vi "Main.vi"(10 "COM port name":refnum<visa-resource-name>, 11 "Module Admin":refnum<class "Delacor_lib_QMH_Cloneable Module Admin.lvclass">) -> ()   [LabVIEW 2018, in "CE14_v2.lvlib"]
doc: "This template is based off of the Queued Message Handler design pattern and the Queued Message Handler project template that ships with LabVIEW.\n\nThe main difference is that the queue is private to this module and communication between modules is performed via Broadcast and Request events.\n\nRequest events are wrapped in public API methods and are handled in the Event Handling Loop (EHL) of this VI. Any module can register for Broadcast events sent by this module. The EHL generates messages based on user interface actions.\n\nThe Message Handling Loop (MHL) processes messages generated by the EHL, or by other messages. The messages are string values, so new messages can be added easily to the Message Cases case structure in the MHL. Each message cluster can also provide an optional value for Message Data, which is a variant that can be converted to whatever message-specific data is required.\n_____\nBased on DQMH Project Template 6.0.0.91."
uses:
  CE14_v2.lvlib
  <vilib>/Delacor/Delacor QMH/Libraries/Cloneable Module Admin_class/Delacor_lib_QMH_Cloneable Module Admin.lvclass
  C:/Program Files (x86)/National Instruments/LabVIEW 2018/vi.lib/Delacor/Delacor QMH/Libraries/Module Admin_class/Delacor_lib_QMH_Module Admin.lvclass
  <vilib>/Delacor/Delacor QMH/Libraries/Message Queue_class/Delacor_lib_QMH_Message Queue.lvclass/Delacor_lib_QMH_Message Queue.ctl
  Module Data--cluster.ctl
  <vilib>/Delacor/Delacor QMH/Libraries/Cloneable Module Admin_class/Delacor_lib_QMH_Cloneable Module Admin.lvclass/Delacor_lib_QMH_Cloneable Module Admin.ctl
  Stop Argument--cluster.ctl
  <vilib>/Delacor/Delacor QMH/Libraries/Module Admin_class/Delacor_lib_QMH_Module Admin.lvclass/Delacor_lib_QMH_Module Admin.ctl
  CE14.CheckConnected Argument--cluster.ctl
  CE14.CheckConnected (Reply Payload)--cluster.ctl
  Read AC parameters Argument--cluster.ctl
  Connect to CE14 Argument--cluster.ctl
  <vilib>/Utility/miscctls.llb/LVPointTypeDef.ctl
  Instrument Drivers/LVdriver_CE14(eMIC)/type defs/CE14.data.ctl
  <vilib>/Delacor/Delacor QMH/Libraries/Message Queue_class/Delacor_lib_QMH_Enqueue Message (Single).vi
  <vilib>/Delacor/Delacor QMH/Libraries/Cloneable Module Admin_class/Delacor_lib_QMH_Get Module ID.vi
  <vilib>/Delacor/Delacor QMH/Libraries/Module Admin_class/Delacor_lib_QMH_Get External Launch.vi
  <vilib>/Utility/error.llb/Error Cluster From Error Code.vi
  <vilib>/ErrorRing/Error Ring.xnode
  <vilib>/Delacor/Delacor QMH/Libraries/Message Queue_class/Delacor_lib_QMH_Message Queue.lvclass
  Instrument Drivers/LVdriver_CE14(eMIC)/CE14_eMIC.lvlib
panel:
  out "Frequency":dbl
  out "connected":bool
  out "error out":errorcluster
  out "Status":string
  in  "Simulate EHL Error":bool
  in  "Simulate MHL Error":bool
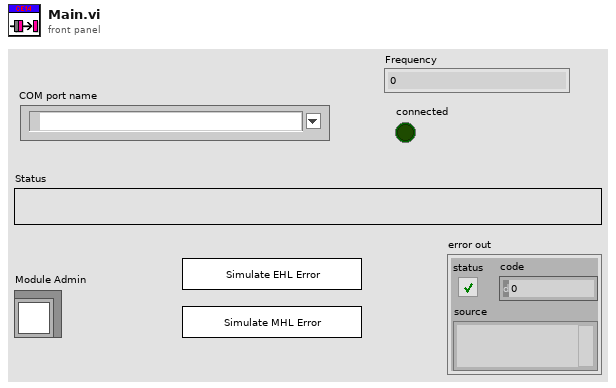
[diagram p1: front panel]
types:
  T1 = typedef "CE14_v2.lvlib/Request Events--cluster.ctl" = cluster{"Stop Module":refnum<user-event>, "Show Panel":refnum<user-event>, "Hide Panel":refnum<user-event>, "Show Diagram":refnum<user-event>, "Get Module Execution Status":refnum<user-event>, "CE14.CheckConnected":refnum<user-event>, "Read AC parameters":refnum<user-event>, "Connect to CE14":refnum<user-event>, "Stop helper loop":refnum<user-event>, "Start Helper Loop":refnum<user-event>}
  T2 = typedef "CE14_v2.lvlib/Module Data--cluster.ctl" = cluster{"Status":string, "VISA resource name":refnum<visa-resource-name>, "connected":bool}
  T3 = enum32{"invalid lock state", "Not Locked", "Locked (No Password)", "Password-protected"}
  T4 = typedef "CE14_v2.lvlib/Stop Argument--cluster.ctl" = cluster{"Module ID":i32, "Origin":string, "Exit via Stop Module Req?":bool, "Wait for Module to stop?":bool}
  T5 = typedef "CE14_v2.lvlib/CE14.CheckConnected Argument--cluster.ctl" = cluster{"Module ID":i32, "Wait Notifier":refnum<notifier>, "wait for reply":bool}
  T6 = typedef "CE14_v2.lvlib/Read AC parameters Argument--cluster.ctl" = cluster{"Module ID":i32, "Boolean":bool}
  T7 = typedef "CE14_v2.lvlib/Connect to CE14 Argument--cluster.ctl" = cluster{"Module ID":i32, "Boolean":bool}
  T8 = typedef "LVPointTypeDef.ctl" = cluster{"Horizontal":i16, "Vertical":i16}
  T9 = enum32{"Invalid", "Standard", "Closed", "Hidden", "Minimized", "Maximized"}
  T10 = typedef "CE14_v2.lvlib/CE14.CheckConnected (Reply Payload)--cluster.ctl" = cluster{"Success":bool, "CE14.CheckConnected_error":errorcluster}
  T11 = typedef "CE14_eMIC.lvlib/CE14.data.ctl" = cluster{"string":string, "float":dbl, "Name":string}
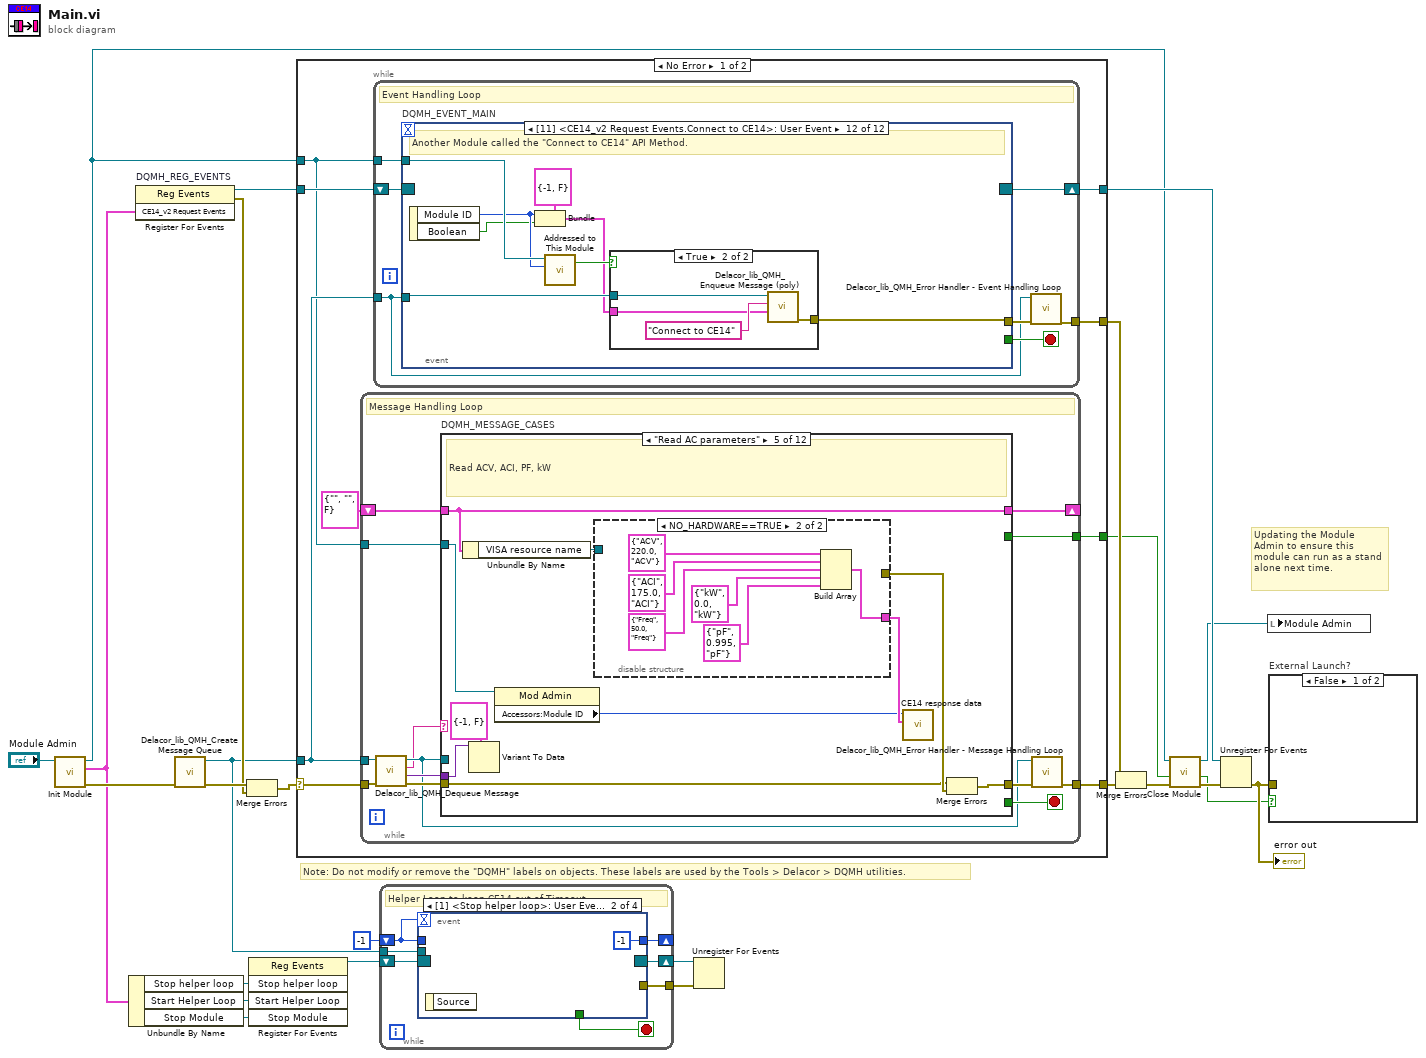
[diagram p0: block diagram]
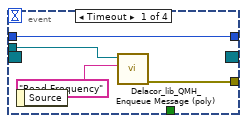
[diagram p2: hidden frame]
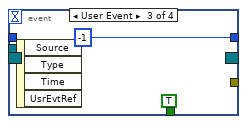
[diagram p3: hidden frame]
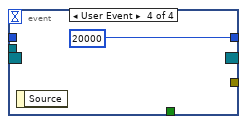
[diagram p4: hidden frame]
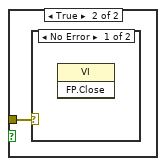
[diagram p5: hidden frame]
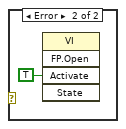
[diagram p6: hidden frame]
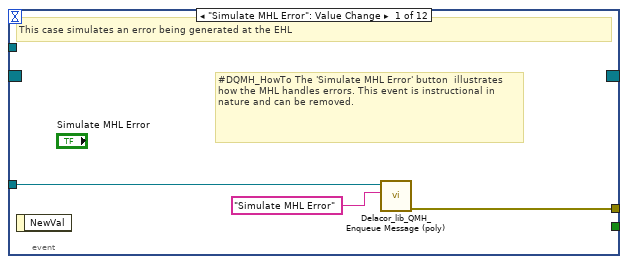
[diagram p7: hidden frame]
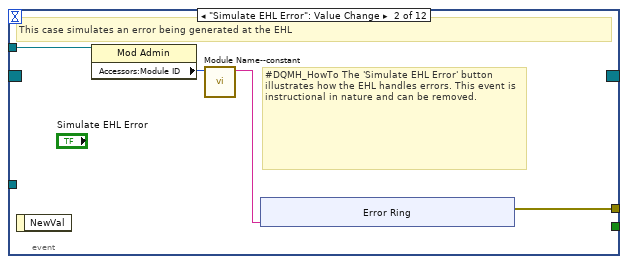
[diagram p8: hidden frame]
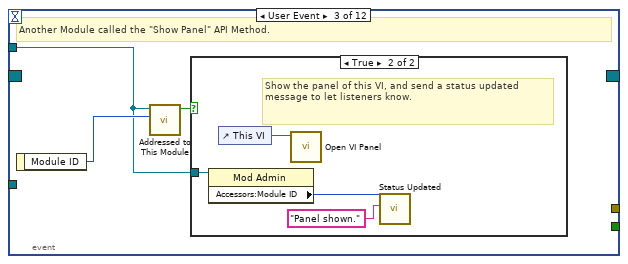
[diagram p9: hidden frame]
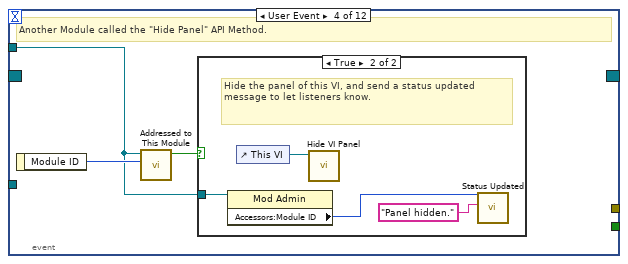
[diagram p11: hidden frame]
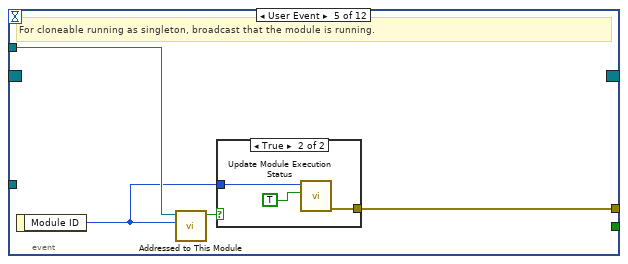
[diagram p13: hidden frame]
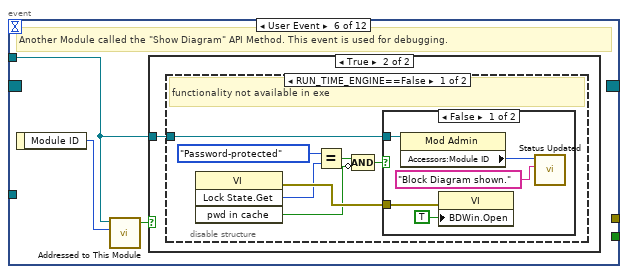
[diagram p15: hidden frame]
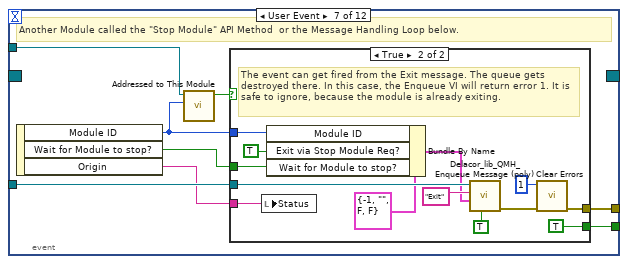
[diagram p19: hidden frame]
diagram:
  # "Note: Do not modify or remove the \"DQMH\" labels on objects. These labels are used by the Tools > Delacor > DQMH utilities."
  # "Updating the Module Admin to ensure this module can run as a stand alone next time."
  n1 = call "Init Module.vi"("Cloneable Module Admin in"="Module Admin") -> ("error out"=w22:errorcluster, "CE14_v2 Request Events"=w8:T1, "Cloneable Module Admin out"=w14:refnum<class "Delacor_lib_QMH_Cloneable Module Admin.lvclass">)  [unwired: 8 in]
  n2 = Unbundle By Name(w8) -> ("Stop helper loop"=w5:refnum<user-event>, "Start Helper Loop"=w4:refnum<user-event>, "Stop Module"=w3:refnum<user-event>)
  n3 = register-events "DQMH_REG_EVENTS"(w8) -> (reference out=w10:refnum<event-registration>, error out=w17:errorcluster)  [unwired: 2 in]
  n4 = call <vilib>:"Delacor_lib_QMH_Create Message Queue.vi"("error in"=w22) -> ("error out"=w19:errorcluster, "Message Queue"=w9:refnum<class "Delacor_lib_QMH_Message Queue.lvclass">)  [unwired: 9 in]
  n5 = Merge Errors(w19, w17) -> (w18:errorcluster)
  n6 = register-events(w5, w4, w3) -> (reference out=w7:refnum<event-registration>)  [unwired: 2 in, 1 out]
  n7 = case shown="No Error" w18 {
    selector: w18 -> [w32 w345]
    tunnel: [w34 w344] -> w23
    tunnel: [w31 w352] -> w16
    tunnel: w10 -> [w29 w352]
    tunnel: w9 -> [w28 w343]
    tunnel: [w33 _] -> w24
    tunnel: w14 -> [w27 w348]
    tunnel: [w26 _] -> w12
    frame No Error {
      n8 = while {
        tunnel: w28 -> [w168]
        shift-right: [w173] -> _
        shift-left: T2 {"Status"="", "VISA resource name"="", "connected"=FALSE} ("Data Cluster") -> [w174]
        tunnel: w32 -> [w169]
        tunnel: [w175] -> w34
        tunnel: w27 -> [w171]
        tunnel: [w170] -> w26
        stop <- w172 stop-if-true
        # "Message Handling Loop"
        n9 = call-dynamic "Delacor_lib_QMH_Dequeue Message.vi"("error in"=w169, "Message Queue in"=w168) -> ("error out"=w166:errorcluster, "Message Data"=w167:variant, "Message"=w164:string, "Message Queue out"=w165:refnum<class "Delacor_lib_QMH_Message Queue.lvclass">)  [unwired: 6 in]
        n10 = case "DQMH_MESSAGE_CASES" shown="\"Read AC parameters\"" w164 {
          selector: w164 -> [_ _ _ _ _ _ _ _ _ _ _ w331]
          tunnel: [w195 w199 w205 w217 w231 w266 w274 w276 w284 w299 w322 w333] -> w176
          tunnel: w174 -> [w179 w200 w203 w220 w237 w268 w275 w277 w283 w297 w313 w332]
          tunnel: [w188 w200 w204 w220 w237 w268 w275 w277 w283 w297 w313 w332] -> w173
          tunnel: [_ _ _ _ _ _ _ _ _ _ w320 _] -> w172
          tunnel: w167 -> [_ _ w209 w227 w239 _ _ _ w282 _ w318 _]
          tunnel: w171 -> [w184 _ _ w216 w233 _ _ _ w281 w295 w308 w329]
          tunnel: [_ _ _ _ _ _ _ _ _ _ w316 _] -> w170
          tunnel: w166 -> [_ w199 w201 w218 w230 w265 w274 w276 _ _ _ _]
          tunnel: w165 -> [_ _ _ _ _ _ _ _ w278 _ w311 _]
          frame "Initialize" {
            w181 = "Initial Message" ("Initial Message")
            # "Initialize - Any operation that needs to be done before the module can receive messages. Synchronize Caller Events.vi will inform Start Module.vi that the module has launched and is ready to receive messages. Module Did Init.vi will broadcast that the module initialized."
            n11 = call "Synchronize Caller Events.vi"("Module Admin"=w184) -> ("error out"=w196:errorcluster, "Module Admin out"=w183:refnum<class "Delacor_lib_QMH_Cloneable Module Admin.lvclass">)  [unwired: 9 in]
            n12 = property class="Mod Admin"(reference=w183) -> ("Accessors:Module ID"=w186:i32, "Accessors:External Launch"=w185:bool)  [unwired: 1 in, 2 out]
            n13 = property on="Pane" class="Pane"("Origin"=T8 {"Horizontal"=0, "Vertical"=0}) -> ()  [unwired: 2 in, 2 out]
            n14 = Bundle By Name(cluster=w179, "VISA resource name"="COM port name") -> (w180:T2)
            n15 = call "Module Name--constant.vi"("Module ID"=w186) -> ("Module Name"=w192:string)  [unwired: 10 in]
            n16 = property class="VI"("Front Panel.Title"=w192) -> (reference out=w194:refnum<vi>, error out=w198:errorcluster)  [unwired: 2 in]
            n17 = Select(t=T9."Hidden" ("State"), s=w185, f=T9."Standard" ("State")) -> (s? t:f=w189:T9)
            n18 = invoke class="VI" method="FP.Open"(reference=w194, error in=w198, "State"=w189) -> (reference out=w193:refnum<vi>, error out=w197:errorcluster)  [unwired: 2 in, 3 out]
            n19 = call "Module Name--constant.vi"("Module ID"=w186) -> ("Module Name"=w187:string)  [unwired: 10 in]
            n20 = Bundle By Name(cluster=w180, "Status"=w181) -> (w188:T2)
            n21 = invoke class="VI" method="FP.Center"(reference=w193, error in=w197) -> ()  [unwired: 1 in, 3 out]
            n22 = call "Module Did Init.vi"("error in (no error)"=w196, "Initialized?"=TRUE, "Origin"=w187, "Module ID"=w186) -> ("error out"=w195:errorcluster)  [unwired: 7 in]
            "Status" <- w181
          }
          frame "---Module Specific---", Default {
            # "Separator -- The following cases handle messages specific to this Module."
          }
          frame "Connect to CE14" {
            # "Open COM and ShakeHand"
            n23 = Unbundle By Name(w203) -> ("VISA resource name"=w207:refnum<visa-resource-name>)
            n24 = Variant To Data(type=T7 {"Module ID"=-1, "Boolean"=FALSE} ("Connect to CE14 Argument"), Variant=w209) -> ()  [unwired: 1 in, 2 out]
            n25 = disable-structure shown="NO_HARDWARE==TRUE" {
              disable-tunnel: w207 -> [w212 _]
              disable-tunnel: [w211 _] -> w206
              disable-tunnel: [w210 TRUE] -> w202
              frame condition #0 {
                n26 = call "CE14.open handshake(subVI).vi"("VISA resource name"=w212) -> ("error out"=w211:errorcluster, "success"=w210:bool)  [unwired: 7 in, 2 out]
              }
              frame condition #1 (active) {
              }
            }
            "connected" <- w202
            n27 = Bundle By Name(cluster=w203, "connected"=w202) -> (w204:T2)
            n28 = Merge Errors(w201, w206) -> (w205:errorcluster)
          }
          frame "CE14.CheckConnected" {
            # "Open port and do shake hand produces"
            n29 = Unbundle By Name(w220) -> ("connected"=w219:bool)
            n30 = Variant To Data(type=T5 {"Module ID"=-1, "Wait Notifier"=refnum, "wait for reply"=FALSE} ("CE14.ShakeHand Argument"), Variant=w227) -> (data=w225:T5)  [unwired: 1 in, 1 out]
            n31 = Unbundle By Name(w225) -> ("Wait Notifier"=w224:refnum<notifier>, "wait for reply"=w223:bool)
            n32 = Bundle By Name(cluster=T10 {"Success"=FALSE, "CE14.CheckConnected_error"={"status"=FALSE, "code"=0, "source"=""}} ("CE14.ShakeHand (Reply Payload)"), "Success"=w219) -> (w222:T10)
            n33 = case shown="True" w223 {
              tunnel: w224 -> [_ w229]
              tunnel: w222 -> [_ w228]
              frame False {
              }
              frame True {
                n34 = Send Notification(notification=w228, notifier=w229) -> ()  [unwired: 1 in, 2 out]
              }
            }
            n35 = property class="Mod Admin"(reference=w216) -> ("Accessors:Module ID"=w215:i32)  [unwired: 1 in, 2 out]
            n36 = call "Start Helper Loop.vi"("Module ID"=w215) -> ("error out"=w214:errorcluster)  [unwired: 10 in]
            n37 = Merge Errors(w218, w214) -> (w217:errorcluster)
          }
          frame "Read AC parameters" {
            # "Read ACV, ACI, PF, kW"
            n38 = Unbundle By Name(w237) -> ("VISA resource name"=w236:refnum<visa-resource-name>)
            n39 = Variant To Data(type=T6 {"Module ID"=-1, "Boolean"=FALSE} ("Read AC parameters Argument"), Variant=w239) -> ()  [unwired: 1 in, 2 out]
            n40 = property class="Mod Admin"(reference=w233) -> ("Accessors:Module ID"=w232:i32)  [unwired: 1 in, 2 out]
            n41 = disable-structure shown="NO_HARDWARE==TRUE" {
              disable-tunnel: w236 -> [w256 _]
              disable-tunnel: [w246 _] -> w235
              disable-tunnel: [w245 w257] -> w234
              frame condition #0 {
                w240 = u32 100 ("milliseconds to wait(100)")
                n42 = call "CE14. Read_Voltage(subVI).vi"("milliseconds to wait(100)"=w240, "VISA resource name"=w256) -> ("error out"=w244:errorcluster, "data out"=w250:T11, "VISA resource name out"=w255:refnum<visa-resource-name>)  [unwired: 6 in, 1 out]
                n43 = call "CE14. Read_Current(subVI).vi"("error in (no error)"=w244, "milliseconds to wait(100)"=w240, "VISA resource name"=w255) -> ("error out"=w243:errorcluster, "dataout"=w251:T11, "VISA resource name out"=w254:refnum<visa-resource-name>)  [unwired: 5 in, 1 out]
                n44 = call "CE14. Read_Freq(subVI).vi"("error in (no error)"=w243, "milliseconds to wait(100)"=w240, "VISA resource name"=w254) -> ("error out"=w242:errorcluster, "data out"=w249:T11, "VISA resource name out"=w253:refnum<visa-resource-name>)  [unwired: 5 in, 1 out]
                n45 = call "CE14. Read_kW(subVI).vi"("error in (no error)"=w242, "milliseconds to wait(100)"=w240, "VISA resource name"=w253) -> ("error out"=w241:errorcluster, "data out"=w248:T11, "VISA resource name out"=w252:refnum<visa-resource-name>)  [unwired: 5 in, 1 out]
                n46 = call "CE14. Read_PowerFactor(subVI).vi"("error in (no error)"=w241, "milliseconds to wait(100)"=w240, "VISA resource name"=w252) -> ("error out"=w246:errorcluster, "data out"=w247:T11)  [unwired: 5 in, 2 out]
                n47 = Build Array(w247, w248, w249, w251, w250) -> (w245:T11[])
              }
              frame condition #1 (active) {
                n48 = Build Array(T11 {"string"="ACV", "float"=220.0, "Name"="ACV"} ("data out"), T11 {"string"="ACI", "float"=175.0, "Name"="ACI"} ("data out"), T11 {"string"="Freq", "float"=50.0, "Name"="Freq"} ("data out"), T11 {"string"="kW", "float"=0.0, "Name"="kW"} ("data out"), T11 {"string"="pF", "float"=0.995, "Name"="pF"} ("data out")) -> (w257:T11[])
              }
            }
            n49 = call "CE14 response data.vi"("Array"=w234, "Module ID"=w232) -> ()  [unwired: 9 in, 1 out]
            n50 = Merge Errors(w230, w235) -> (w231:errorcluster)
          }
          frame "Read Frequency" {
            n51 = Unbundle By Name(w268) -> ("VISA resource name"=w267:refnum<visa-resource-name>)
            n52 = disable-structure shown="NO_HARDWARE==TRUE" {
              disable-tunnel: w267 -> [w272 _]
              disable-tunnel: [w271 _] -> w264
              disable-tunnel: [w269 50.0 ("float")] -> w263
              frame condition #0 {
                n53 = call "CE14. Read_Freq(subVI).vi"("VISA resource name"=w272) -> ("error out"=w271:errorcluster, "data out"=w270:T11)  [unwired: 7 in, 2 out]
                n54 = Unbundle By Name(w270) -> ("float"=w269:dbl)
              }
              frame condition #1 (active) {
              }
            }
            "Frequency" <- w263
            n55 = Merge Errors(w265, w264) -> (w266:errorcluster)
          }
          frame "---Copy This Frame---" {
            # "Duplicate this frame when creating new messages.  Change this comment in the duplicated frame to describe this message."
          }
          frame "---Exit and Error Handling---" {
            # "Separator - the following cases handle errors and exit messages."
          }
          frame "Error" {
            # "Error - Check the error message data and respond accordingly. This message is sent by the \"Error Handler\" VIs at the end of each loop in this application."
            n56 = property class="Mod Admin"(reference=w281) -> ("Accessors:External Launch"=w280:bool, "Accessors:Module ID"=w279:i32)  [unwired: 1 in, 2 out]
            n57 = Variant To Data(type=errorcluster {"status"=FALSE, "code"=0, "source"=""} ("error constant"), Variant=w282) -> (data=w288:errorcluster, error out=w286:errorcluster)  [unwired: 1 in]
            n58 = call "Error Reported.vi"("Error"=w288, "Module ID"=w279) -> ()  [unwired: 9 in, 1 out]
            n59 = case shown="False" w280 {
              tunnel: [w293 _] -> w285
              tunnel: w288 -> [w292 _]
              tunnel: w278 -> [w289 _]
              frame False {
                # "If the module is running standalone, then pop up an error dialog and call the \"Exit\" message."
                n60 = call <vilib>:"Simple Error Handler.vi"("error in (no error)"=w292) -> ()  [unwired: 4 in, 5 out]
                n61 = call-poly <vilib>:"Delacor_lib_QMH_Enqueue Message (poly).vi"("Priority Message? (F)"=TRUE, "Message"="Exit", "Message Queue in"=w289) -> ("error out"=w293:errorcluster)  [unwired: 7 in, 1 out]
              }
              frame True {
                # "If the module was launched externally, calling the Error Reported broadcast VI is the only action performed by the \"Error\" message. The module's caller can then process the error appropriately."
              }
            }
            n62 = Merge Errors(w286, w285) -> (w284:errorcluster)
            n63 = local write "error out"(w284) -> ()
          }
          frame "Simulate MHL Error" {
            # "#DQMH_HowTo The 'Simulate MHL Error' button  illustrates how the MHL handles errors. This event is instructional in nature and can be removed."
            # "Simulate an error occurring at the MHL"
            n64 = property class="Mod Admin"(reference=w295) -> ("Accessors:Module ID"=w296:i32)  [unwired: 1 in, 2 out]
            n65 = call "Module Name--constant.vi"("Module ID"=w296) -> ("Module Name"=w294:string)  [unwired: 10 in]
            n66 = xnode "Error Ring"("parameter 0"=w294) -> ("error out"=w298:errorcluster)
            n67 = Merge Errors(w298) -> (w299:errorcluster)
          }
          frame "Exit" {
            w319 = 91  # 91: not all Exit messages will have an argument
            w320 = TRUE  # Stop the VI
            # "Release the message queue reference"
            # "Exit - Exit the application."
            n68 = Variant To Data(type=T4 {"Module ID"=-1, "Origin"="", "Exit via Stop Module Req?"=FALSE, "Wait for Module to stop?"=FALSE} ("Stop Argument"), Variant=w318) -> (data=w315:T4, error out=w321:errorcluster)  [unwired: 1 in]
            n69 = disable-structure shown="NO_HARDWARE==TRUE" {
              disable-tunnel: w313 -> [w327 _]
              disable-tunnel: [w325 _] -> w312
              frame condition #0 {
                n70 = Unbundle By Name(w327) -> ("VISA resource name"=w326:refnum<visa-resource-name>)
                n71 = call "CE14 Close Connection (SubVI).vi"("VISA Refnum in"=w326) -> ("error out"=w325:errorcluster)  [unwired: 10 in]
              }
              frame condition #1 (active) {
              }
            }
            n72 = call <vilib>:"Clear Errors.vi"("error in (no error)"=w321, "specific error code to clear (0: all)"=w319) -> ("error out"=w324:errorcluster)  [unwired: 4 in, 1 out]
            n73 = control-ref of="This VI"() -> (w314:refnum<vi>)
            n74 = property class="Mod Admin"(reference=w308) -> ("Accessors:Module ID"=w307:i32)  [unwired: 1 in, 2 out]
            n75 = call-dynamic "Delacor_lib_QMH_Release Message Queue.vi"("error in"=w324, "Message Queue"=w311) -> ("error out"=w323:errorcluster)  [unwired: 9 in]
            n76 = call "Handle Exit.vi"("error in (no error)"=w312, "Stop Argument"=w315, "Module Admin in"=w308, "VI reference"=w314) -> ("error out"=w310:errorcluster, "Wait for Stop?"=w316:bool)  [unwired: 6 in]
            n77 = call "Stop helper loop.vi"("error in"=w310, "Module ID"=w307) -> ("error out"=w309:errorcluster)  [unwired: 9 in]
            n78 = Merge Errors(w323, w309) -> (w322:errorcluster)
          }
          frame "example" {
            # "'Default' case only runs if there is a message that isn't defined in any of the other cases.  Output a programming error."
            n79 = property class="Mod Admin"(reference=w329) -> ("Accessors:Module ID"=w328:i32)  [unwired: 1 in, 2 out]
            n80 = call "Module Name--constant.vi"("Module ID"=w328) -> ("Module Name"=w330:string)  [unwired: 10 in]
            n81 = xnode "Error Ring"("parameter 0"=w331, "parameter 1"=w330) -> ("error out"=w334:errorcluster)
            n82 = Merge Errors(w334) -> (w333:errorcluster)
          }
        }
        n83 = call-dynamic "Delacor_lib_QMH_Error Handler - Message Handling Loop.vi"("error in"=w176, "Message Queue in"=w165) -> ("dup error in"=w175:errorcluster)  [unwired: 8 in, 1 out]
      }
      n84 = while {
        tunnel: w28 -> [w35]
        shift-right: [w38] -> w31
        shift-left: w29 -> [w39]
        tunnel: [w40] -> w33
        tunnel: w27 -> [w36]
        stop <- w37 stop-if-true
        # "Event Handling Loop"
        n85 = event "DQMH_EVENT_MAIN" shown="[11] <CE14_v2 Request Events.Connect to CE14>: User Event" {
          selector: w39 -> [_ _ _ _ _ _ _ _ _ _ _ _]
          dyn-events: [_ _ _ _ _ _ _ _ _ _ _ _] -> w38
          timeout: _ -> [_ _ _ _ _ _ _ _ _ _ _ _]
          tunnel: [_ _ _ _ _ _ w97 _ _ _ _ _] -> w37
          tunnel: w35 -> [w43 _ _ _ _ _ w99 w115 w132 w144 w151 w159]
          tunnel: [w44 w48 _ _ w73 _ w100 w118 w124 w137 w149 w152] -> w41
          tunnel: w36 -> [_ w47 w56 w63 w71 w77 w93 w116 w130 w142 _ w157]
          event "Simulate MHL Error": Value Change {
            # "#DQMH_HowTo The 'Simulate MHL Error' button  illustrates how the MHL handles errors. This event is instructional in nature and can be removed."
            # "This case simulates an error being generated at the EHL"
            n86 = event-data() -> ()  [unwired: 1 in, 1 out]
            n87 = call-poly <vilib>:"Delacor_lib_QMH_Enqueue Message (poly).vi"("Message"="Simulate MHL Error", "Message Queue in"=w43) -> ("error out"=w44:errorcluster)  [unwired: 8 in, 1 out]
          }
          event "Simulate EHL Error": Value Change {
            # "#DQMH_HowTo The 'Simulate EHL Error' button  illustrates how the EHL handles errors. This event is instructional in nature and can be removed."
            # "This case simulates an error being generated at the EHL"
            n88 = event-data() -> ()  [unwired: 1 in, 1 out]
            n89 = property class="Mod Admin"(reference=w47) -> ("Accessors:Module ID"=w46:i32)  [unwired: 1 in, 2 out]
            n90 = call "Module Name--constant.vi"("Module ID"=w46) -> ("Module Name"=w45:string)  [unwired: 10 in]
            n91 = xnode "Error Ring"("parameter 0"=w45) -> ("error out"=w48:errorcluster)
          }
          event User Event {
            # "Another Module called the \"Show Panel\" API Method."
            n92 = event-data() -> ("Module ID"=w57:i32)  [unwired: 1 in]
            n93 = call "Addressed to This Module.vi"("Module ID from Argument"=w57, "Module Admin"=w56) -> ("Addressed to this instance?"=w58:bool)  [unwired: 8 in, 1 out]
            n94 = case shown="True" w58 {
              tunnel: w56 -> [_ w60]
              frame False {
              }
              frame True {
                # "Show the panel of this VI, and send a status updated message to let listeners know."
                n95 = property class="Mod Admin"(reference=w60) -> ("Accessors:Module ID"=w59:i32)  [unwired: 1 in, 2 out]
                n96 = control-ref of="This VI"() -> (w62:refnum<vi>)
                n97 = call "Open VI Panel.vi"("VI"=w62) -> ()  [unwired: 10 in, 1 out]
                n98 = call "Status Updated.vi"("Status"="Panel shown." ("format string"), "Module ID"=w59) -> ()  [unwired: 9 in, 1 out]
              }
            }
          }
          event User Event {
            # "Another Module called the \"Hide Panel\" API Method."
            n99 = event-data() -> ("Module ID"=w64:i32)  [unwired: 1 in]
            n100 = call "Addressed to This Module.vi"("Module ID from Argument"=w64, "Module Admin"=w63) -> ("Addressed to this instance?"=w65:bool)  [unwired: 8 in, 1 out]
            n101 = case shown="True" w65 {
              tunnel: w63 -> [_ w67]
              frame False {
              }
              frame True {
                # "Hide the panel of this VI, and send a status updated message to let listeners know."
                n102 = property class="Mod Admin"(reference=w67) -> ("Accessors:Module ID"=w66:i32)  [unwired: 1 in, 2 out]
                n103 = control-ref of="This VI"() -> (w69:refnum<vi>)
                n104 = call "Hide VI Panel.vi"("VI"=w69) -> ()  [unwired: 10 in, 1 out]
                n105 = call "Status Updated.vi"("Status"="Panel hidden." ("format string"), "Module ID"=w66) -> ()  [unwired: 9 in, 1 out]
              }
            }
          }
          event User Event {
            # "For cloneable running as singleton, broadcast that the module is running."
            n106 = event-data() -> ("Module ID"=w70:i32)  [unwired: 1 in]
            n107 = call "Addressed to This Module.vi"("Module ID from Argument"=w70, "Module Admin"=w71) -> ("Addressed to this instance?"=w72:bool)  [unwired: 8 in, 1 out]
            n108 = case shown="True" w72 {
              tunnel: [_ w76] -> w73
              tunnel: w70 -> [_ w75]
              frame False {
              }
              frame True {
                n109 = call "Update Module Execution Status.vi"("Running?"=TRUE, "Module ID"=w75) -> ("error out"=w76:errorcluster)  [unwired: 9 in]
              }
            }
          }
          event User Event {
            # "Another Module called the \"Show Diagram\" API Method. This event is used for debugging."
            n110 = event-data() -> ("Module ID"=w78:i32)  [unwired: 1 in]
            n111 = call "Addressed to This Module.vi"("Module ID from Argument"=w78, "Module Admin"=w77) -> ("Addressed to this instance?"=w79:bool)  [unwired: 8 in, 1 out]
            n112 = case shown="True" w79 {
              tunnel: w77 -> [_ w80]
              frame False {
              }
              frame True {
                n113 = disable-structure shown="RUN_TIME_ENGINE==False" {
                  disable-tunnel: w80 -> [w81 _]
                  frame condition #0 (active) {
                    # "functionality not available in exe"
                    n114 = invoke class="VI" method="Lock State.Get"() -> (error out=w87:errorcluster, "Get Lock State"=w86:T3, "pwd in cache"=w83:bool)  [unwired: 4 in, 1 out]
                    n115 = Equal?(x=T3."Password-protected", y=w86) -> (x = y?=w84:bool)
                    n116 = Compound Arithmetic op=AND(w84, invert w83) -> (w82:bool)
                    n117 = case shown="False" w82 {
                      tunnel: w87 -> [w92 _]
                      tunnel: w81 -> [w89 _]
                      frame False {
                        n118 = property class="Mod Admin"(reference=w89) -> ("Accessors:Module ID"=w88:i32)  [unwired: 1 in, 2 out]
                        n119 = property class="VI"(error in=w92, "BDWin.Open"=TRUE ("Block Diagram Window:Open")) -> ()  [unwired: 1 in, 2 out]
                        n120 = call "Status Updated.vi"("Status"="Block Diagram shown." ("format string"), "Module ID"=w88) -> ()  [unwired: 9 in, 1 out]
                      }
                      frame True {
                        # "Password-protected VI, and the password is not in the cache. Do not show the diagram."
                      }
                    }
                  }
                  frame condition #1 {
                  }
                }
              }
            }
          }
          event User Event {
            # "Another Module called the \"Stop Module\" API Method  or the Message Handling Loop below."
            n121 = event-data() -> ("Module ID"=w94:i32, "Wait for Module to stop?"=w96:bool, "Origin"=w95:string)  [unwired: 1 in]
            n122 = call "Addressed to This Module.vi"("Module ID from Argument"=w94, "Module Admin"=w93) -> ("Addressed to this instance?"=w98:bool)  [unwired: 8 in, 1 out]
            n123 = case shown="True" w98 {
              tunnel: [_ w112] -> w100
              tunnel: w99 -> [_ w108]
              tunnel: [_ TRUE] -> w97
              tunnel: w96 -> [_ w103]
              tunnel: w94 -> [_ w105]
              tunnel: w95 -> [_ w101]
              frame False {
              }
              frame True {
                # "The event can get fired from the Exit message. The queue gets destroyed there. In this case, the Enqueue VI will return error 1. It is safe to ignore, because the module is already exiting."
                n124 = local write "Status"(w101) -> ()
                n125 = Bundle By Name(cluster=T4 {"Module ID"=-1, "Origin"="", "Exit via Stop Module Req?"=FALSE, "Wait for Module to stop?"=FALSE} ("Stop Argument"), "Module ID"=w105, "Exit via Stop Module Req?"=TRUE, "Wait for Module to stop?"=w103) -> (w102:T4)
                n126 = call-poly <vilib>:"Delacor_lib_QMH_Enqueue Message (poly).vi"("Priority Message? (F)"=TRUE, "Message Data"=w102, "Message"="Exit", "Message Queue in"=w108) -> ("error out"=w113:errorcluster)  [unwired: 6 in, 1 out]
                n127 = call <vilib>:"Clear Errors.vi"("error in (no error)"=w113, "specific error code to clear (0: all)"=1) -> ("error out"=w112:errorcluster)  [unwired: 4 in, 1 out]
              }
            }
          }
          event Panel Close? {
            w117 = TRUE  # Discard the event, the MHL is responsible for closing and stopping this VI.
            # "Hide the panel or send the 'Exit' message if the user clicks the 'X' on the module main VI panel."
            n128 = event-data() -> ()  [unwired: 1 in, 1 out]
            n129 = property class="Mod Admin"(reference=w116) -> ("Accessors:External Launch"=w114:bool)  [unwired: 1 in, 2 out]
            n130 = case shown="False" w114 {
              tunnel: w115 -> [_ w122]
              tunnel: [_ w123] -> w118
              frame True {
                # "If externally launched, clicking the 'X' hides the panel, but doesn't close it."
                n131 = control-ref of="This VI"() -> (w119:refnum<vi>)
                n132 = call "Hide VI Panel.vi"("VI"=w119) -> ()  [unwired: 10 in, 1 out]
              }
              frame False {
                # "If run as a stand-alone VI, clicking the panel 'X' stops the VI."
                n133 = call-poly <vilib>:"Delacor_lib_QMH_Enqueue Message (poly).vi"("Priority Message? (F)"=TRUE, "Message"="Exit", "Message Queue in"=w122) -> ("error out"=w123:errorcluster)  [unwired: 7 in, 1 out]
              }
            }
            n134 = event-data("Discard?"=w117) -> ()  [unwired: 1 in, 1 out]
          }
          event User Event {
            # "Another Module called the \"CE14.ShakeHand\" API Method."
            n135 = event-data() -> ("Module ID"=w127:i32, "Wait Notifier"=w126:refnum<notifier>, "wait for reply"=w125:bool)  [unwired: 1 in]
            n136 = Bundle(cluster=T5 {"Module ID"=-1, "Wait Notifier"=refnum, "wait for reply"=FALSE} ("CE14.ShakeHand Argument"), "Module ID"=w127, "Wait Notifier"=w126, "wait for reply"=w125) -> (w128:T5)
            n137 = call "Addressed to This Module.vi"("Module ID from Argument"=w127, "Module Admin"=w130) -> ("Addressed to this instance?"=w131:bool)  [unwired: 8 in, 1 out]
            n138 = case shown="True" w131 {
              tunnel: w132 -> [_ w136]
              tunnel: w128 -> [_ w134]
              tunnel: [_ w133] -> w124
              frame False {
              }
              frame True {
                n139 = call-poly <vilib>:"Delacor_lib_QMH_Enqueue Message (poly).vi"("Message Data"=w134, "Message"="CE14.CheckConnected", "Message Queue in"=w136) -> ("error out"=w133:errorcluster)  [unwired: 7 in, 1 out]
              }
            }
          }
          event User Event {
            # "Another Module called the \"Read AC parameters\" API Method."
            n140 = event-data() -> ("Module ID"=w139:i32, "Boolean"=w138:bool)  [unwired: 1 in]
            n141 = Bundle(cluster=T6 {"Module ID"=-1, "Boolean"=FALSE} ("Read AC parameters Argument"), "Module ID"=w139, "Boolean"=w138) -> (w140:T6)
            n142 = call "Addressed to This Module.vi"("Module ID from Argument"=w139, "Module Admin"=w142) -> ("Addressed to this instance?"=w143:bool)  [unwired: 8 in, 1 out]
            n143 = case shown="False" w143 {
              tunnel: w144 -> [_ w148]
              tunnel: w140 -> [_ w145]
              tunnel: [_ w146] -> w137
              frame False {
              }
              frame True {
                n144 = call-poly <vilib>:"Delacor_lib_QMH_Enqueue Message (poly).vi"("Message Data"=w145, "Message"="Read AC parameters", "Message Queue in"=w148) -> ("error out"=w146:errorcluster)  [unwired: 7 in, 1 out]
              }
            }
          }
          event Timeout {
            # "No use"
            # "Keep CE14's connection"
            n145 = event-data() -> ()  [unwired: 1 in, 1 out]
            n146 = call-poly <vilib>:"Delacor_lib_QMH_Enqueue Message (poly).vi"("Message"="Read Frequency", "Message Queue in"=w151) -> ("error out"=w149:errorcluster)  [unwired: 8 in, 1 out]
          }
          event User Event {
            # "Another Module called the \"Connect to CE14\" API Method."
            n147 = event-data() -> ("Module ID"=w154:i32, "Boolean"=w153:bool)  [unwired: 1 in]
            n148 = Bundle(cluster=T7 {"Module ID"=-1, "Boolean"=FALSE} ("Connect to CE14 Argument"), "Module ID"=w154, "Boolean"=w153) -> (w155:T7)
            n149 = call "Addressed to This Module.vi"("Module ID from Argument"=w154, "Module Admin"=w157) -> ("Addressed to this instance?"=w158:bool)  [unwired: 8 in, 1 out]
            n150 = case shown="True" w158 {
              tunnel: w159 -> [_ w163]
              tunnel: w155 -> [_ w161]
              tunnel: [_ w160] -> w152
              frame False {
              }
              frame True {
                n151 = call-poly <vilib>:"Delacor_lib_QMH_Enqueue Message (poly).vi"("Message Data"=w161, "Message"="Connect to CE14", "Message Queue in"=w163) -> ("error out"=w160:errorcluster)  [unwired: 7 in, 1 out]
              }
            }
          }
        }
        n152 = call-dynamic "Delacor_lib_QMH_Error Handler - Event Handling Loop.vi"("error in"=w41, "Message Queue in"=w35) -> ("dup error in"=w40:errorcluster)  [unwired: 8 in, 1 out]
      }
    }
    frame Error {
      n153 = call "Synchronize Caller Events.vi"("Module Admin"=w348) -> ("Module Admin out"=w347:refnum<class "Delacor_lib_QMH_Cloneable Module Admin.lvclass">)  [unwired: 9 in, 1 out]
      n154 = property class="Mod Admin"(reference=w347) -> ("Accessors:Module ID"=w346:i32)  [unwired: 1 in, 2 out]
      n155 = call-dynamic "Delacor_lib_QMH_Release Message Queue.vi"("error in"=w345, "Message Queue"=w343) -> ("error out"=w344:errorcluster)  [unwired: 9 in]
      n156 = call "Module Name--constant.vi"("Module ID"=w346) -> ("Module Name"=w351:string)  [unwired: 10 in]
      n157 = Format Into String(format string="An error occurred during initialization. %s is no longer running.", w351) -> (resulting string=w349:string)  [unwired: 2 in, 1 out]
      n158 = call "Error Reported.vi"("Additional Information"=w349, "Error"=w344, "Module ID"=w346) -> ()  [unwired: 8 in, 1 out]
    }
  }
  n159 = while {
    shift-right: [w357] -> _
    shift-left: -1 -> [w358]
    tunnel: w9 -> [w356]
    shift-right: [w355] -> w6
    shift-left: w7 -> [w359]
    tunnel: [w353] -> w1
    stop <- w354 stop-if-true
    # "Helper Loop to keep CE14 out of Timeout"
    n160 = event shown="[1] <Stop helper loop>: User Event" {
      selector: w359 -> [_ _ _ _]
      dyn-events: [_ _ _ _] -> w355
      timeout: w358 -> [_ _ _ _]
      tunnel: [_ _ TRUE _] -> w354
      tunnel: w358 -> [w363 _ _ _]
      tunnel: [w363 -1 -1 20000] -> w357
      tunnel: w356 -> [w362 _ _ _]
      tunnel: [w360 _ _ _] -> w353
      event Timeout {
        n161 = event-data() -> ()  [unwired: 1 in, 1 out]
        n162 = call-poly <vilib>:"Delacor_lib_QMH_Enqueue Message (poly).vi"("Message"="Read Frequency", "Message Queue in"=w362) -> ("error out"=w360:errorcluster)  [unwired: 8 in, 1 out]
      }
      event User Event {
        n163 = event-data() -> ()  [unwired: 1 in, 1 out]
      }
      event User Event {
        n164 = event-data() -> ()  [unwired: 1 in, 4 out]
      }
      event User Event {
        n165 = event-data() -> ()  [unwired: 1 in, 1 out]
      }
    }
  }
  n166 = Unregister For Events(event registration refnum=w6, error in=w1) -> ()  [unwired: 1 out]
  n167 = Merge Errors(w24, w23) -> (w25:errorcluster)
  n168 = call "Close Module.vi"("error in"=w25, "Wait for stop?"=w12, "Module Admin in"=w14) -> ("error out"=w21:errorcluster, "External Launch"=w11:bool, "Module Admin out"=w13:refnum<class "Delacor_lib_QMH_Cloneable Module Admin.lvclass">)  [unwired: 6 in]
  n169 = Unregister For Events(event registration refnum=w16, error in=w21) -> (error out=w20:errorcluster)
  "error out" <- w20
  n170 = local write "Module Admin"(w13) -> ()
  n171 = case "External Launch?" shown="False" w11 {
    tunnel: w20 -> [_ w368]
    frame False {
    }
    frame True {
      n172 = case shown="No Error" w368 {
        frame No Error {
          n173 = invoke class="VI" method="FP.Close"() -> ()  [unwired: 3 in, 3 out]
        }
        frame Error {
          n174 = invoke class="VI" method="FP.Open"("Activate"=TRUE ("Activate?")) -> ()  [unwired: 4 in, 5 out]
        }
      }
    }
  }
